vi "Get Ref Phase Value.vi"(8 "error in (no error)":errorcluster, 11 "VISA resource name":refnum<visa-resource-name>) -> (0 "error out":errorcluster, 2 "Phase Value":dbl format="%.4f", 3 "VISA resource name out":refnum<visa-resource-name>)   [LabVIEW 2013, in "Fluke 5XXX Series Multicalibrators.lvlib"]
doc: "If two Calibrators are synchronized using 10 MHz IN/OUT, returns the phase difference between the primary channel on the Calibrator and the sync pulse on the 10 MHz IN or OUT terminal.\n\nNote:\n\nThis VI is available only for instrument model 5520A."
uses:
  Fluke 5XXX Series Multicalibrators.lvlib
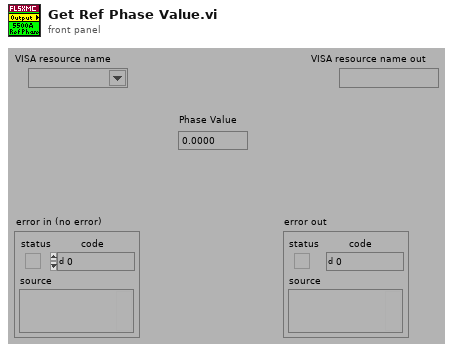
[diagram p1: front panel]
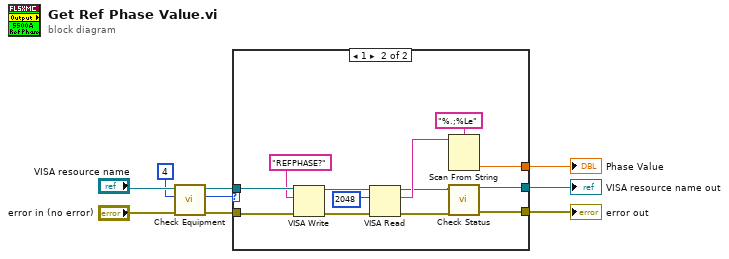
[diagram p0: block diagram]
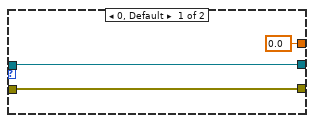
[diagram p2: hidden frame]
diagram:
  n1 = call "Check Equipment.vi"("error in (no error)"="error in (no error)", "Bit Mask"=4 ("Numeric"), "VISA resource name"="VISA resource name") -> ("error out"=w9:errorcluster, "Present?"=w8:u32, "VISA resource name out"=w7:refnum<visa-resource-name>)  [unwired: 6 in]
  n2 = case shown="1" w8 {
    tunnel: w9 -> [w12 w24]
    tunnel: w7 -> [w10 w23]
    tunnel: [w12 w25] -> w4
    tunnel: [0.0 w14] -> w3
    tunnel: [w10 w13] -> w1
    frame 0, Default {
    }
    frame 1 {
      n3 = VISA Write(VISA resource name=w23, write buffer="REFPHASE?", error in (no error)=w24) -> (VISA resource name out=w20:refnum<visa-resource-name>, error out=w19:errorcluster)  [unwired: 1 out]
      n4 = VISA Read(VISA resource name=w20, byte count=u32 2048 ("byte count (0)"), error in (no error)=w19) -> (VISA resource name out=w15:refnum<visa-resource-name>, read buffer=w16:string, error out=w17:errorcluster)  [unwired: 1 out]
      n5 = Scan From String(format string="%.;%Le", input string=w16) -> (output 1=w14:dbl)  [unwired: 3 in, 3 out]
      n6 = call "Check Status.vi"("VISA resource name"=w15, "error in (no error)"=w17) -> ("VISA resource name out"=w13:refnum<visa-resource-name>, "error out"=w25:errorcluster)  [unwired: 12 in]
    }
  }
  "Phase Value" <- w3
  "VISA resource name out" <- w1
  "error out" <- w4
